vi "setTrigger.vi"(8 "error in (no error)":errorcluster, 9 "Args":string[](array[string]), 10 "Command":string, 11 "TektronixDPOSimple in":refnum<class "TektronixDPO.lvclass">) -> (0 "error out":errorcluster, 2 "new commands":string, 3 "TektronixDPOSimple out":refnum<class "TektronixDPO.lvclass">)   [LabVIEW 2013, in "TektronixDPO.lvclass"]
doc: "Set the speficied Trigger subproperty value, and update the CVT"
uses:
  TektronixDPO.lvclass
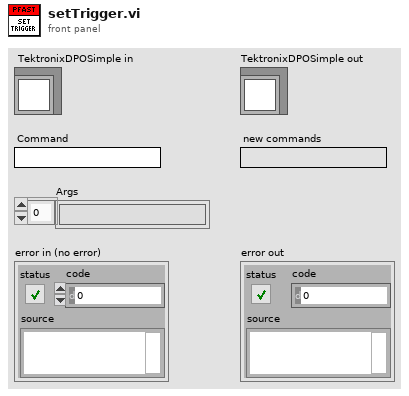
[diagram p1: front panel]
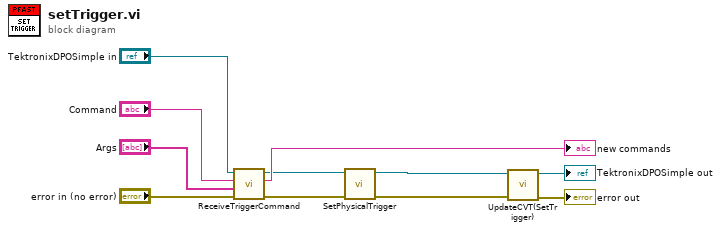
[diagram p0: block diagram]
diagram:
  n1 = call "ReceiveTriggerCommand.vi"("error in (no error)"="error in (no error)", "Args"="Args", "Command"="Command", "TektronixDPOSimple in"="TektronixDPOSimple in") -> ("error out"=w5:errorcluster, "new commands"=→"new commands":string, "TektronixDPOSimple out"=w3:refnum<class "TektronixDPO.lvclass">)  [unwired: 5 in]
  n2 = call "SetPhysicalTrigger.vi"("error in (no error)"=w5, "TektronixDPO in"=w3) -> ("error out"=w4:errorcluster, "TektronixDPO out"=w2:refnum<class "TektronixDPO.lvclass">)  [unwired: 8 in]
  n3 = call "UpdateCVT(SetTrigger).vi"("error in (no error)"=w4, "TektronixDPO in"=w2) -> ("error out"=→"error out":errorcluster, "TektronixDPO out"=→"TektronixDPOSimple out":refnum<class "TektronixDPO.lvclass">)  [unwired: 8 in]
